vi "parameter.vi"(1 "default":fxp<+/-,32,16>, 2 "set":bool, 3 "new":fxp<+/-,32,16>) -> (0 "value":fxp<+/-,32,16>)   [LabVIEW 2018]
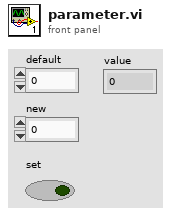
[diagram p1: front panel]
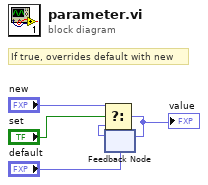
[diagram p0: block diagram]
diagram:
  # "If true, overrides default with new"
  n1 = feedback #1("default") -> (w2:fxp<+/-,32,16>)
  n2 = Select(t="new", s="set", f=w2) -> (s? t:f=w5:fxp<+/-,32,16>)
  "value" <- w5
  n3 = feedback-in #1(w5) -> ()
